vi "MCListbox Event - Key Down QuestionMark.vi"(8 "Error In":errorcluster, 9 "Key Down?":bool, 11 "CtlRef":refnum<vi>) -> (0 "Error Out":errorcluster)   [LabVIEW 2013]
panel:
  out "Selected MCListBox":string
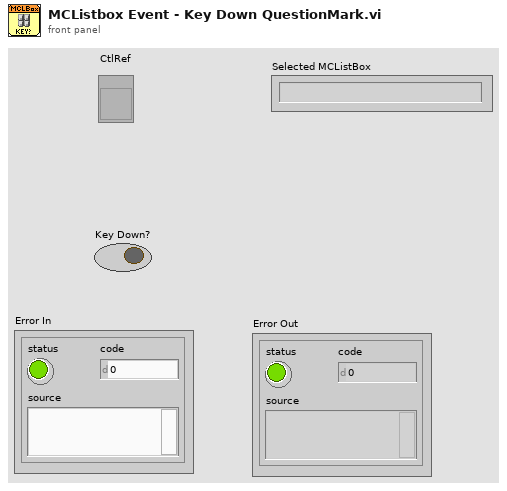
[diagram p1: front panel]
types:
  T1 = typedef "LVRowAndColumnTypeDef.ctl" = cluster{"Row":i32, "Column":i32}
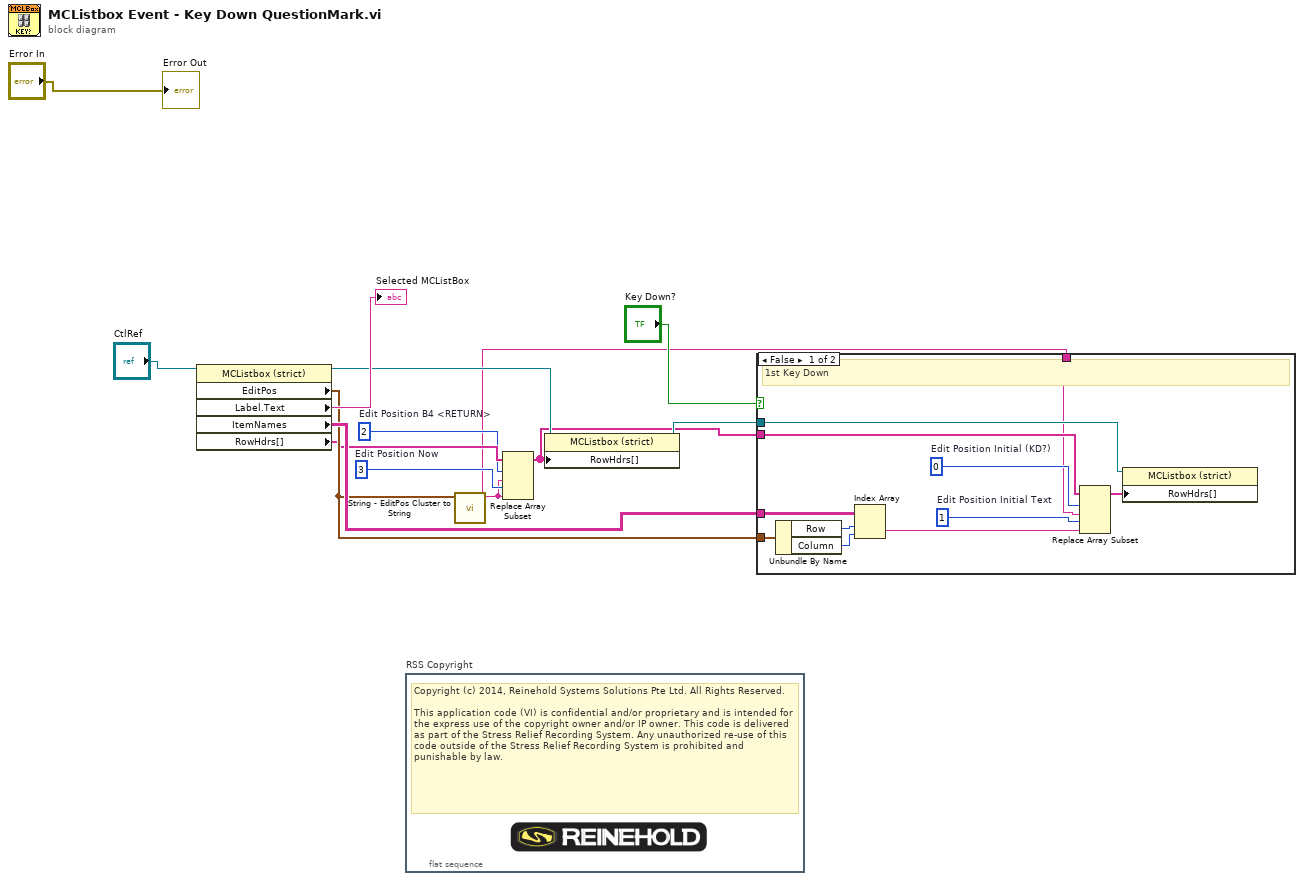
[diagram p0: block diagram]
diagram:
  w5 = 3  # Edit Position Now
  w6 = 2  # Edit Position B4 <RETURN>
  n1 = property on="Property Node" class="MCListbox (strict)"(reference="CtlRef") -> (reference out=w4:refnum<vi>, "EditPos"=w8:T1, "Label.Text"=→"Selected MCListBox":string, "ItemNames"=w10:string[][], "RowHdrs[]"=w7:string[])  [unwired: 1 in, 1 out]
  n2 = flat-sequence "RSS Copyright" {
    frame #0 {
      # "Copyright (c) 2014, Reinehold Systems Solutions Pte Ltd. All Rights Reserved.\n\nThis application code (VI) is confidential and/or proprietary and is intended for the express use of the copyright owner and/or IP owner. This code is delivered as part of the Stress Relief Recording System. Any unauthorized re-use of this code outside of the Stress Relief Recording System is prohibited and punishable by law."
    }
  }
  n3 = call "String - EditPos Cluster to String.vi"("EditPos"=w8) -> ("result string"=w3:string)  [unwired: 10 in]
  n4 = Replace Array Subset(array=w7, new element #1=w3, index #1=w6, new element #2=w3, index #2=w5) -> (w1:string[])
  n5 = property class="MCListbox (strict)"(reference=w4, "RowHdrs[]"=w1) -> (reference out=w2:refnum<vi>)  [unwired: 1 in, 1 out]
  n6 = case shown="False" "Key Down?" {
    tunnel: w8 -> [w20 _]
    tunnel: w10 -> [w23 _]
    tunnel: w2 -> [w21 _]
    tunnel: w1 -> [w19 _]
    tunnel: w3 -> [w14 _]
    frame False {
      w15 = 1  # Edit Position Initial Text
      w18 = 0  # Edit Position Initial (KD?)
      # "1st Key Down"
      n7 = Unbundle By Name(w20) -> ("Row"=w24:i32, "Column"=w22:i32)
      n8 = Index Array(array=w23, index (row)=w24, index (col)=w22) -> (element=w16:string)
      n9 = Replace Array Subset(array=w19, new element #1=w14, index #1=w18, new element #2=w16, index #2=w15) -> (w17:string[])
      n10 = property class="MCListbox (strict)"(reference=w21, "RowHdrs[]"=w17) -> ()  [unwired: 1 in, 2 out]
    }
    frame True {
    }
  }
  "Error Out" <- "Error In"
